vi "Begin.vi"(8 "error in":errorcluster) -> (0 "error out":errorcluster)   [LabVIEW 2014]
doc: "Called before other user functions, this VI is expected to open initial I/O refnums, load in file data, and do all program initialization. Notice that the <B>error out</B> terminal is simply used for data flow. Wiring it to other structures or subVIs ensures that this VI runs first."
uses:
  <vilib>/Rock Robotics/SystemInterfaces/DIO/FPGA_DIOChannel.ctl
  <vilib>/Rock Robotics/SystemInterfaces/DIO/FPGA_DIORelayChannel.ctl
  <vilib>/Rock Robotics/WPI/Relay/WPI_RelayDirection.ctl
  <vilib>/Rock Robotics/SystemInterfaces/AI/FPGA_AIChannel.ctl
  <vilib>/Rock Robotics/WPI/SafetyOutput/WPI_SafetyOutputConfigMenu.ctl
  <vilib>/Rock Robotics/WPI/Solenoid/WPI_SolenoidChannel.ctl
  <vilib>/Rock Robotics/WPI/Joystick/WPI_JoystickDeviceEnum.ctl
  <vilib>/Rock Robotics/WPI/Compressor/WPI_CompressorGetSetRefNum.vi
  <vilib>/Rock Robotics/WPI/RobotDrive/WPI_RobotDriveOpen4MotorWithCANTalonSRX.vi
  <vilib>/Rock Robotics/WPI/MotorControl/WPI_MotorControlOpenCANTalonSRX.vi
  <vilib>/Rock Robotics/WPI/Solenoid/WPI_SolenoidOpenSingle.vi
  Robot Global Data.vi
  navX-MXP Library/navX-MXP IMU.lvlib
  navX-MXP Library/SERIAL/IO/NI WPI/WPI_SerialPort_USB.ctl
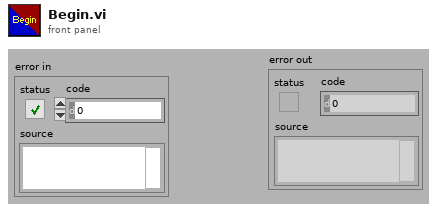
[diagram p1: front panel]
types:
  T1 = typedef "WPI_RelayDirection.ctl" = enum16{"Both directions", "Forward only", "Reverse only"}
  T2 = typedef "FPGA_DIORelayChannel.ctl" = enum8{"Relay 0", "Relay 1", "Relay 2", "Relay 3", "Invalid"}
  T3 = typedef "FPGA_DIOChannel.ctl" = enum8{"DIO 0", "DIO 1", "DIO 2", "DIO 3", "DIO 4", "DIO 5", "DIO 6", "DIO 7", "DIO 8", "DIO 9", "DIO MXP 0", "DIO MXP 1", "DIO MXP 2", "DIO MXP 3", "DIO MXP 4", "DIO MXP 5", "DIO MXP 6", "DIO MXP 7", "DIO MXP 8", "DIO MXP 9", "DIO MXP 10", "DIO MXP 11", "DIO MXP 12", "DIO MXP 13", "DIO MXP 14", "DIO MXP 15", "Invalid"}
  T4 = typedef "WPI_SolenoidChannel.ctl" = enum8{"Solenoid 0", "Solenoid 1", "Solenoid 2", "Solenoid 3", "Solenoid 4", "Solenoid 5", "Solenoid 6", "Solenoid 7", "Invalid"}
  T5 = typedef "WPI_SolenoidDevRef.ctl" = cluster{"DevStatus":errorcluster, "Pneumatics Control Module":u8, "Forward Solenoid Channel":T4, "Reverse Solenoid Channel":T4}
  T6 = cluster{"String Potentiometer":dbl, "Setpoint":dbl, "Level":sgl}
  T7 = typedef "WPI_CompressorDevRef.ctl" = cluster{"DevStatus":errorcluster, "Pneumatics Control Module":u8}
  T8 = typedef "navX-MXP IMU.lvlib/WPI_SerialPort_USB.ctl" = enum16{"Onboard RS-232", "MXP TTL", "USB"}
  T9 = typedef "navX-MXP IMU.lvlib/navX SPI DevRef.ctl" = cluster{"SPIDevRef":T10, "Board Information":T13, "Status":T14, "Offsets":cluster{"Yaw":dbl, "Quat W":dbl, "Quat X":dbl, "Quat Y":dbl, "Quat Z":dbl}, "Update Rate (4Hz-60Hz)":u8, "refnum name":string, "error":errorcluster}
  T10 = typedef "WPI_SPIDevRef.ctl" = cluster{"DevStatus":errorcluster, "Handle":i32, "Controller":T11, "SPI Bus":T12}
  T11 = typedef "FPGA_TypedefDigitalModule.ctl" = enum16{"Controller 1"}
  T12 = typedef "spi_bus.ctl" = enum16{"SPI On-Board, CS0", "SPI On-Board, CS1", "SPI On-Board, CS2", "SPI On-Board, CS3", "SPI MXP", "Invalid"}
  T13 = typedef "navX-MXP IMU.lvlib/navX Board Information.ctl" = cluster{"WhoAmI (50 | 0x32)":u8, "Board Revision":u8, "Firmware Major Version":u8, "Firmware Minor Version":u8}
  T14 = typedef "navX-MXP IMU.lvlib/navX Status Data.ctl" = cluster{"Update Rate Hz":u8, "Accelerometer Full-Scale Range":u8, "Gyro Full-Scale Range":u16, "NAVX_OP_STATUS":T15, "NAVX_CAL_STATUS":T16, "NAVX_SELFTEST_STATUS":u8, "NAVX_SENSOR_STATUS":T17}
  T15 = typedef "navX-MXP IMU.lvlib/navX NAVX_OP_STATUS.ctl" = u8
  T16 = typedef "navX-MXP IMU.lvlib/navX NAVX_CAL_STATUS.ctl" = u8
  T17 = typedef "navX-MXP IMU.lvlib/navX NAVX_SENSOR_STATUS.ctl" = cluster{"MOVING":bool, "YAW_STABLE":bool, "MAG_DISTURBANCE":bool, "ALTITUDE_VALID":bool, "SEALEVEL_PRESS_SET":bool, "FUSED_HEADING_VALID":bool}
  T18 = typedef "navX-MXP IMU.lvlib/navX Serial DevRef.ctl" = cluster{"SerialPortRef":T19, "Board Information":T13, "Status":T14, "Offsets":cluster{"Yaw":dbl, "Quat W":dbl, "Quat X":dbl, "Quat Y":dbl, "Quat Z":dbl}, "Update Rate (4Hz-60Hz)":u8, "Nav6Mode (YPR)":T20, "refnum name":string, "error":errorcluster}
  T19 = typedef "WPI_SerialPortRef.ctl" = cluster{"DevStatus":errorcluster, "Serial Port Name":refnum<visa-resource-name>}
  T20 = typedef "navX-MXP IMU.lvlib/navX Serial Mode.ctl" = enum16{"YPR", "Gyro", "Quaternion"}
  T21 = typedef "WPI_DigitalInputDevRef.ctl" = cluster{"DevStatus":errorcluster, "DIO Channel":T3, "Controller":T11}
  T22 = typedef "WPI_RelayDevRef.ctl" = cluster{"DevStatus":errorcluster, "Relay Channel":T2, "Controller":T11, "Relay Direction":T1}
  T23 = typedef "FPGA_AIChannel.ctl" = enum8{"AI 0", "AI 1", "AI 2", "AI 3", "AI MXP 0", "AI MXP 1", "AI MXP 2", "AI MXP 3", "Invalid"}
  T24 = typedef "WPI_AnalogChannelDevRef.ctl" = cluster{"DevStatus":errorcluster, "Controller":T25, "Analog Channel":T23}
  T25 = typedef "FPGA_TypedefAnalogModule.ctl" = enum16{"Controller 1"}
  T26 = typedef "WPI_SafetyOutputConfigMenu.ctl" = enum16{"Enable", "Disable"}
  T27 = typedef "WPI_RobotDriveDevRef.ctl" = cluster{"DevStatus":errorcluster, "Motors[]":T28[], "Square Inputs":bool, "Max Output":dbl}
  T28 = typedef "WPI_MotorControlDeviceRef.ctl" = cluster{"DeviceStatus":errorcluster, "Type":T29, "PWM":cluster{"Controller":T11, "PWM Channel":T30, "DeadBand":T31}, "CAN":cluster{"Device Number":u8, "Control Mode":T32, "Semaphore":T33, "Max Vout":dbl, "TalonSRX Control Mode":T34}, "Invert":bool, "TransformRef":T35, "InvTransformRef":T35}
  T29 = typedef "WPI_MotorControlType.ctl" = enum16{"PWM", "CAN", "CANTalonSRX"}
  T30 = typedef "FPGA_DIOPWMChannel.ctl" = enum8{"PWM 0", "PWM 1", "PWM 2", "PWM 3", "PWM 4", "PWM 5", "PWM 6", "PWM 7", "PWM 8", "PWM 9", "PWM MXP 0", "PWM MXP 1", "PWM MXP 2", "PWM MXP 3", "PWM MXP 4", "PWM MXP 5", "PWM MXP 6", "PWM MXP 7", "PWM MXP 8", "PWM MXP 9", "Invalid"}
  T31 = typedef "WPI_PWMDeadband.ctl" = cluster{"Name":string, "maxPositivePwm":i32, "minPositivePwm":i32, "centerPwm":i32, "maxNegativePwm":i32, "minNegativePwm":i32, "angularRange":u16}
  T32 = typedef "WPI_CANJaguar_ControlMode.ctl" = enum8{"Percent VBus", "Current", "Speed", "Position", "Voltage"}
  T33 = typedef "Semaphore RefNum" = refnum<k1>
  T34 = typedef "WPI_CANTalonSRX_APIControlMode.ctl" = enum8{"Percent VBus", "Speed", "Position", "Slave", "Unchanged / Invalid"}
  T35 = typedef "WPI_PWMTransform_ConPane.ctl" = refnum<vi>
  T36 = typedef "WPI_JoystickDeviceEnum.ctl" = enum16{"USB 0", "USB 1", "USB 2", "USB 3", "USB 4", "USB 5"}
  T37 = typedef "WPI_JoystickDevRef.ctl" = cluster{"Device":T36}
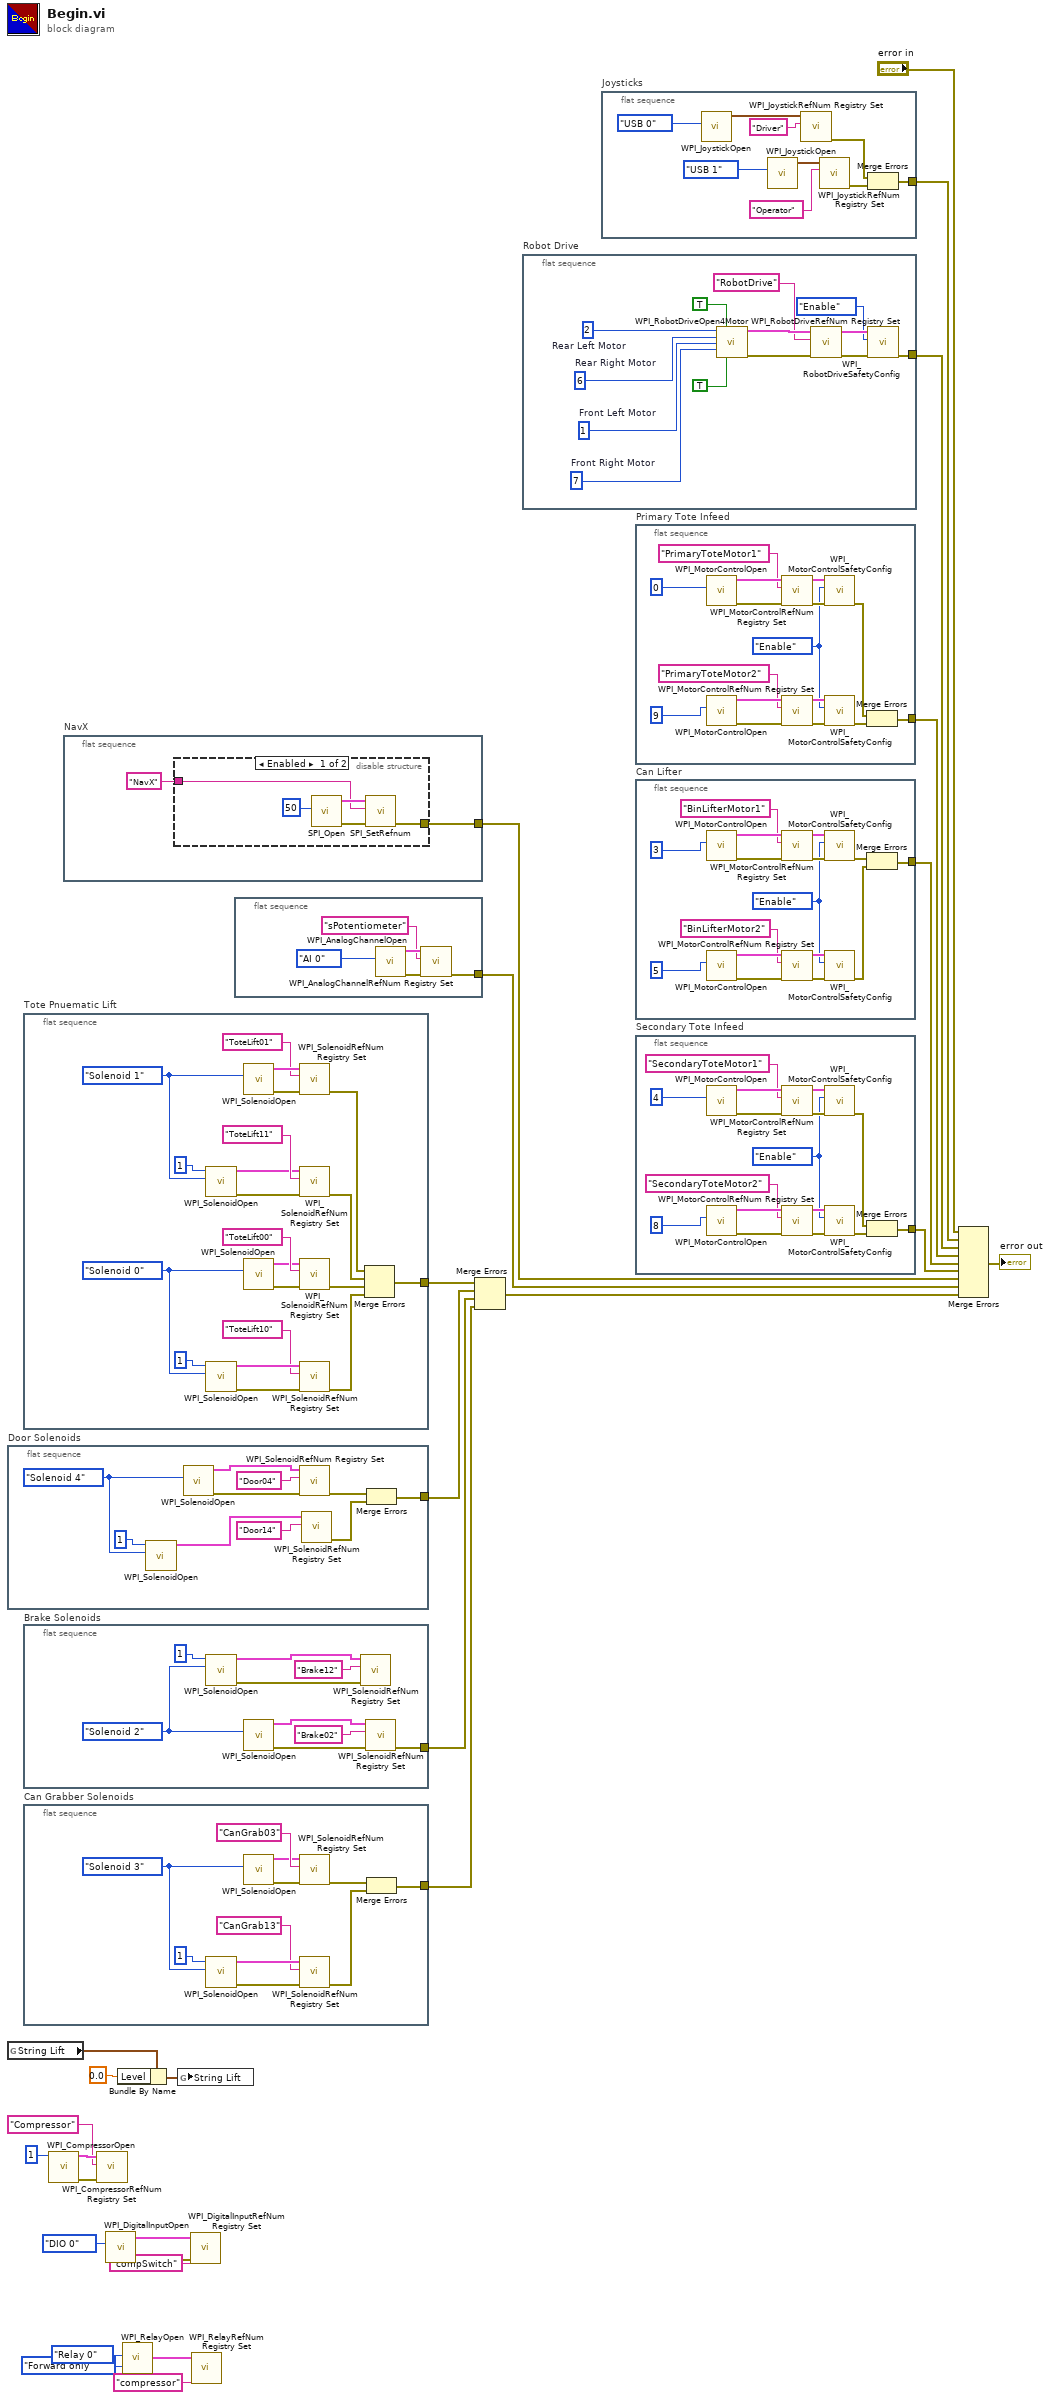
[diagram p0: block diagram]
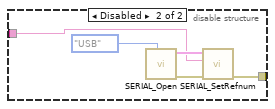
[diagram p2: hidden frame]
diagram:
  n1 = flat-sequence "Door Solenoids" {
    tunnel: [w30] -> w17
    frame #0 {
      w36 = WPI_SolenoidChannel."Solenoid 4" ("Reverse Solenoid Channel")
      n2 = call-poly <vilib>:"WPI_SolenoidOpen.vi"("Solenoid Channel"=w36, "Pneumatics Control Module (0)"=u8 1) -> ("SolenoidDevRef"=w35:T5)  [unwired: 8 in, 1 out]
      n3 = call-poly <vilib>:"WPI_SolenoidOpen.vi"("Solenoid Channel"=w36) -> ("error out"=w33:errorcluster, "SolenoidDevRef"=w34:T5)  [unwired: 9 in]
      n4 = call <vilib>:"WPI_SolenoidRefNum Registry Set.vi"("error in (no error)"=w33, "refnum name"="Door04", "SolenoidDevRef"=w34) -> ("error out"=w32:errorcluster)  [unwired: 7 in, 1 out]
      n5 = call <vilib>:"WPI_SolenoidRefNum Registry Set.vi"("refnum name"="Door14", "SolenoidDevRef"=w35) -> ("error out"=w31:errorcluster)  [unwired: 8 in, 1 out]
      n6 = Merge Errors(w32, w31) -> (w30:errorcluster)
    }
  }
  n7 = global read "Robot Global Data.vi" "String Lift"() -> (w15:T6)
  n8 = flat-sequence "Tote Pnuematic Lift" {
    tunnel: [w43] -> w16
    frame #0 {
      w47 = WPI_SolenoidChannel."Solenoid 1" ("Forward Solenoid Channel")
      w54 = WPI_SolenoidChannel."Solenoid 0" ("Forward Solenoid Channel")
      n9 = call-poly <vilib>:"WPI_SolenoidOpen.vi"("Solenoid Channel"=w47, "Pneumatics Control Module (0)"=u8 1) -> ("error out"=w48:errorcluster, "SolenoidDevRef"=w49:T5)  [unwired: 8 in]
      n10 = call-poly <vilib>:"WPI_SolenoidOpen.vi"("Solenoid Channel"=w54, "Pneumatics Control Module (0)"=u8 1) -> ("error out"=w60:errorcluster, "SolenoidDevRef"=w59:T5)  [unwired: 8 in]
      n11 = call-poly <vilib>:"WPI_SolenoidOpen.vi"("Solenoid Channel"=w47) -> ("error out"=w53:errorcluster, "SolenoidDevRef"=w52:T5)  [unwired: 9 in]
      n12 = call-poly <vilib>:"WPI_SolenoidOpen.vi"("Solenoid Channel"=w54) -> ("error out"=w55:errorcluster, "SolenoidDevRef"=w56:T5)  [unwired: 9 in]
      n13 = call <vilib>:"WPI_SolenoidRefNum Registry Set.vi"("error in (no error)"=w53, "refnum name"="ToteLift01", "SolenoidDevRef"=w52) -> ("error out"=w42:errorcluster)  [unwired: 7 in, 1 out]
      n14 = call <vilib>:"WPI_SolenoidRefNum Registry Set.vi"("error in (no error)"=w48, "refnum name"="ToteLift11", "SolenoidDevRef"=w49) -> ("error out"=w41:errorcluster)  [unwired: 7 in, 1 out]
      n15 = call <vilib>:"WPI_SolenoidRefNum Registry Set.vi"("error in (no error)"=w55, "refnum name"="ToteLift00", "SolenoidDevRef"=w56) -> ("error out"=w40:errorcluster)  [unwired: 7 in, 1 out]
      n16 = call <vilib>:"WPI_SolenoidRefNum Registry Set.vi"("error in (no error)"=w60, "refnum name"="ToteLift10", "SolenoidDevRef"=w59) -> ("error out"=w44:errorcluster)  [unwired: 7 in, 1 out]
      n17 = Merge Errors(w42, w41, w40, w44) -> (w43:errorcluster)
    }
  }
  n18 = flat-sequence "Brake Solenoids" {
    tunnel: [w66] -> w18
    frame #0 {
      w62 = WPI_SolenoidChannel."Solenoid 2" ("Reverse Solenoid Channel")
      n19 = call-poly <vilib>:"WPI_SolenoidOpen.vi"("Solenoid Channel"=w62, "Pneumatics Control Module (0)"=u8 1) -> ("error out"=w65:errorcluster, "SolenoidDevRef"=w61:T5)  [unwired: 8 in]
      n20 = call-poly <vilib>:"WPI_SolenoidOpen.vi"("Solenoid Channel"=w62) -> ("error out"=w67:errorcluster, "SolenoidDevRef"=w68:T5)  [unwired: 9 in]
      n21 = call <vilib>:"WPI_SolenoidRefNum Registry Set.vi"("error in (no error)"=w65, "refnum name"="Brake12", "SolenoidDevRef"=w61) -> ()  [unwired: 7 in, 2 out]
      n22 = call <vilib>:"WPI_SolenoidRefNum Registry Set.vi"("error in (no error)"=w67, "refnum name"="Brake02", "SolenoidDevRef"=w68) -> ("error out"=w66:errorcluster)  [unwired: 7 in, 1 out]
    }
  }
  n23 = flat-sequence "Can Grabber Solenoids" {
    tunnel: [w70] -> w19
    frame #0 {
      w79 = WPI_SolenoidChannel."Solenoid 3" ("Reverse Solenoid Channel")
      n24 = call-poly <vilib>:"WPI_SolenoidOpen.vi"("Solenoid Channel"=w79, "Pneumatics Control Module (0)"=u8 1) -> ("error out"=w78:errorcluster, "SolenoidDevRef"=w77:T5)  [unwired: 8 in]
      n25 = call-poly <vilib>:"WPI_SolenoidOpen.vi"("Solenoid Channel"=w79) -> ("error out"=w73:errorcluster, "SolenoidDevRef"=w74:T5)  [unwired: 9 in]
      n26 = call <vilib>:"WPI_SolenoidRefNum Registry Set.vi"("error in (no error)"=w73, "refnum name"="CanGrab03", "SolenoidDevRef"=w74) -> ("error out"=w72:errorcluster)  [unwired: 7 in, 1 out]
      n27 = call <vilib>:"WPI_SolenoidRefNum Registry Set.vi"("error in (no error)"=w78, "refnum name"="CanGrab13", "SolenoidDevRef"=w77) -> ("error out"=w71:errorcluster)  [unwired: 7 in, 1 out]
      n28 = Merge Errors(w72, w71) -> (w70:errorcluster)
    }
  }
  n29 = call <vilib>:"WPI_CompressorOpen.vi"("Pneumatics Control Module (0)"=u8 1) -> ("CompressorDevRef"=w21:T7, "error out"=w22:errorcluster)  [unwired: 13 in]
  n30 = flat-sequence "NavX" {
    tunnel: [w82] -> w11
    frame #0 {
      n31 = disable-structure shown="Enabled" {
        disable-tunnel: [w84 w88] -> w82
        disable-tunnel: "NavX" ("refnum name") -> [w83 w89]
        frame Enabled {
          n32 = call "SPI_Open.vi"("Update Rate (4Hz-60Hz)"=u8 50) -> ("error out"=w86:errorcluster, "navX DevRef"=w85:T9)  [unwired: 8 in, 1 out]
          n33 = call "SPI_SetRefnum.vi"("error in (no error)"=w86, "refnum name"=w83, "navX DevRef"=w85) -> ("error out"=w84:errorcluster)  [unwired: 7 in, 1 out]
        }
        frame Disabled {
          n34 = call "SERIAL_Open.vi"("Serial Port (MXP)"=WPI_SerialPort_USB."USB") -> ("error out"=w92:errorcluster, "navX Ref"=w91:T18)  [unwired: 8 in, 1 out]
          n35 = call "SERIAL_SetRefnum.vi"("error in (no error)"=w92, "refnum name"=w89, "navX DevRef"=w91) -> ("error out"=w88:errorcluster)  [unwired: 7 in, 1 out]
        }
      }
    }
  }
  n36 = call <vilib>:"WPI_CompressorRefNum Registry Set.vi"("error in (no error)"=w22, "refnum name"="Compressor", "CompressorDevRef"=w21) -> ()  [unwired: 7 in, 2 out]
  n37 = call <vilib>:"WPI_DigitalInputOpen.vi"("DIO Channel"=FPGA_DIOChannel."DIO 0") -> ("error out"=w7:errorcluster, "DigitalInputDevRef"=w8:T21)  [unwired: 9 in]
  n38 = Bundle By Name(cluster=w15, "Level"=sgl 0.0) -> (w14:T6)
  n39 = call <vilib>:"WPI_RelayOpen.vi"("Relay Direction"=WPI_RelayDirection."Forward only", "Relay Channel"=FPGA_DIORelayChannel."Relay 0") -> ("RelayDevRef"=w2:T22)  [unwired: 8 in, 1 out]
  n40 = global write "Robot Global Data.vi" "String Lift"(w14) -> ()
  n41 = call <vilib>:"WPI_DigitalInputRefNum Registry Set.vi"("error in (no error)"=w7, "refnum name"="compSwitch", "DigitalInputDevRef"=w8) -> ()  [unwired: 7 in, 2 out]
  n42 = call <vilib>:"WPI_RelayRefNum Registry Set.vi"("refnum name"="compressor", "RelayDevRef"=w2) -> ()  [unwired: 8 in, 2 out]
  n43 = flat-sequence {
    tunnel: [w95] -> w10
    frame #0 {
      n44 = call <vilib>:"WPI_AnalogChannelOpen.vi"("Analog Channel"=FPGA_AIChannel."AI 0") -> ("error out"=w96:errorcluster, "AIDeviceRef"=w97:T24)  [unwired: 9 in]
      n45 = call <vilib>:"WPI_AnalogChannelRefNum Registry Set.vi"("error in (no error)"=w96, "refnum name"="sPotentiometer", "AIDeviceRef"=w97) -> ("error out"=w95:errorcluster)  [unwired: 7 in, 1 out]
    }
  }
  n46 = Merge Errors(w16, w17, w18, w19) -> (w9:errorcluster)
  n47 = flat-sequence "Robot Drive" {
    tunnel: [w100] -> w29
    frame #0 {
      w107 = u8 7  # Front Right Motor
      w108 = u8 1  # Front Left Motor
      w109 = u8 6  # Rear Right Motor
      w110 = u8 2  # Rear Left Motor
      n48 = call-poly <vilib>:"WPI_RobotDriveOpen4Motor.vi"("Rear Left Motor"=w110, "Rear Left Motor Inverted"=TRUE, "Rear Right Motor"=w109, "Front Left Motor"=w108, "Front Right Motor"=w107, "Front Left Motor Inverted"=TRUE) -> ("RobotDriveDevRef"=w106:T27, "error out"=w105:errorcluster)  [unwired: 8 in]
      n49 = call <vilib>:"WPI_RobotDriveRefNum Registry Set.vi"("error in (no error)"=w105, "refnum name"="RobotDrive", "RobotDriveDevRef"=w106) -> ("error out"=w102:errorcluster, "RobotDriveDevRef"=w103:T27)  [unwired: 7 in]
      n50 = call <vilib>:"WPI_RobotDriveSafetyConfig.vi"("error in (no error)"=w102, "mode"=WPI_SafetyOutputConfigMenu."Enable", "RobotDriveDevRef"=w103) -> ("error out"=w100:errorcluster)  [unwired: 7 in, 1 out]
    }
  }
  n51 = flat-sequence "Joysticks" {
    tunnel: [w115] -> w28
    frame #0 {
      n52 = call <vilib>:"WPI_JoystickOpen.vi"("JoystickDevice"=WPI_JoystickDeviceEnum."USB 0") -> ("JoystickDevRef"=w117:T37)  [unwired: 10 in]
      n53 = call <vilib>:"WPI_JoystickOpen.vi"("JoystickDevice"=WPI_JoystickDeviceEnum."USB 1") -> ("JoystickDevRef"=w113:T37)  [unwired: 10 in]
      n54 = call <vilib>:"WPI_JoystickRefNum Registry Set.vi"("refnum name"="Driver", "JoystickDevRef"=w117) -> ("error out"=w116:errorcluster)  [unwired: 8 in, 1 out]
      n55 = call <vilib>:"WPI_JoystickRefNum Registry Set.vi"("refnum name"="Operator", "JoystickDevRef"=w113) -> ("error out"=w111:errorcluster)  [unwired: 8 in, 1 out]
      n56 = Merge Errors(w116, w111) -> (w115:errorcluster)
    }
  }
  n57 = flat-sequence "Primary Tote Infeed" {
    tunnel: [w124] -> w27
    frame #0 {
      w121 = WPI_SafetyOutputConfigMenu."Enable" ("mode")
      n58 = call-poly <vilib>:"WPI_MotorControlOpen.vi"("Device Number"=u8 0) -> ("error out"=w134:errorcluster, "MotorControlDeviceRef"=w133:T28)  [unwired: 9 in]
      n59 = call-poly <vilib>:"WPI_MotorControlOpen.vi"("Device Number"=u8 9 ("Master Device Number")) -> ("error out"=w132:errorcluster, "MotorControlDeviceRef"=w131:T28)  [unwired: 9 in]
      n60 = call <vilib>:"WPI_MotorControlRefNum Registry Set.vi"("error in (no error)"=w134, "refnum name"="PrimaryToteMotor1", "MotorControlDevRef"=w133) -> ("error out"=w129:errorcluster, "MotorControlDevRef"=w130:T28)  [unwired: 7 in]
      n61 = call <vilib>:"WPI_MotorControlRefNum Registry Set.vi"("error in (no error)"=w132, "refnum name"="PrimaryToteMotor2", "MotorControlDevRef"=w131) -> ("error out"=w128:errorcluster, "MotorControlDevRef"=w127:T28)  [unwired: 7 in]
      n62 = call <vilib>:"WPI_MotorControlSafetyConfig.vi"("error in (no error)"=w129, "mode"=w121, "MotorControlDevRef"=w130) -> ("error out"=w126:errorcluster)  [unwired: 7 in, 1 out]
      n63 = call <vilib>:"WPI_MotorControlSafetyConfig.vi"("error in (no error)"=w128, "mode"=w121, "MotorControlDevRef"=w127) -> ("error out"=w125:errorcluster)  [unwired: 7 in, 1 out]
      n64 = Merge Errors(w126, w125) -> (w124:errorcluster)
    }
  }
  n65 = flat-sequence "Can Lifter" {
    tunnel: [w141] -> w26
    frame #0 {
      w138 = WPI_SafetyOutputConfigMenu."Enable" ("mode")
      n66 = call-poly <vilib>:"WPI_MotorControlOpen.vi"("Device Number"=u8 3 ("Master Device Number")) -> ("error out"=w151:errorcluster, "MotorControlDeviceRef"=w150:T28)  [unwired: 9 in]
      n67 = call-poly <vilib>:"WPI_MotorControlOpen.vi"("Device Number"=u8 5 ("Master Device Number")) -> ("error out"=w149:errorcluster, "MotorControlDeviceRef"=w148:T28)  [unwired: 9 in]
      n68 = call <vilib>:"WPI_MotorControlRefNum Registry Set.vi"("error in (no error)"=w151, "refnum name"="BinLifterMotor1", "MotorControlDevRef"=w150) -> ("error out"=w147:errorcluster, "MotorControlDevRef"=w146:T28)  [unwired: 7 in]
      n69 = call <vilib>:"WPI_MotorControlRefNum Registry Set.vi"("error in (no error)"=w149, "refnum name"="BinLifterMotor2", "MotorControlDevRef"=w148) -> ("error out"=w145:errorcluster, "MotorControlDevRef"=w144:T28)  [unwired: 7 in]
      n70 = call <vilib>:"WPI_MotorControlSafetyConfig.vi"("error in (no error)"=w147, "mode"=w138, "MotorControlDevRef"=w146) -> ("error out"=w143:errorcluster)  [unwired: 7 in, 1 out]
      n71 = call <vilib>:"WPI_MotorControlSafetyConfig.vi"("error in (no error)"=w145, "mode"=w138, "MotorControlDevRef"=w144) -> ("error out"=w142:errorcluster)  [unwired: 7 in, 1 out]
      n72 = Merge Errors(w143, w142) -> (w141:errorcluster)
    }
  }
  n73 = flat-sequence "Secondary Tote Infeed" {
    tunnel: [w156] -> w12
    frame #0 {
      w153 = WPI_SafetyOutputConfigMenu."Enable" ("mode")
      n74 = call-poly <vilib>:"WPI_MotorControlOpen.vi"("Device Number"=u8 4) -> ("error out"=w166:errorcluster, "MotorControlDeviceRef"=w165:T28)  [unwired: 9 in]
      n75 = call-poly <vilib>:"WPI_MotorControlOpen.vi"("Device Number"=u8 8 ("Master Device Number")) -> ("error out"=w164:errorcluster, "MotorControlDeviceRef"=w163:T28)  [unwired: 9 in]
      n76 = call <vilib>:"WPI_MotorControlRefNum Registry Set.vi"("error in (no error)"=w166, "refnum name"="SecondaryToteMotor1", "MotorControlDevRef"=w165) -> ("error out"=w161:errorcluster, "MotorControlDevRef"=w162:T28)  [unwired: 7 in]
      n77 = call <vilib>:"WPI_MotorControlRefNum Registry Set.vi"("error in (no error)"=w164, "refnum name"="SecondaryToteMotor2", "MotorControlDevRef"=w163) -> ("error out"=w160:errorcluster, "MotorControlDevRef"=w159:T28)  [unwired: 7 in]
      n78 = call <vilib>:"WPI_MotorControlSafetyConfig.vi"("error in (no error)"=w161, "mode"=w153, "MotorControlDevRef"=w162) -> ("error out"=w158:errorcluster)  [unwired: 7 in, 1 out]
      n79 = call <vilib>:"WPI_MotorControlSafetyConfig.vi"("error in (no error)"=w160, "mode"=w153, "MotorControlDevRef"=w159) -> ("error out"=w157:errorcluster)  [unwired: 7 in, 1 out]
      n80 = Merge Errors(w158, w157) -> (w156:errorcluster)
    }
  }
  n81 = Merge Errors("error in", w28, w29, w27, w26, w12, w11, w10, w9) -> (→"error out":errorcluster)
